vi "DATADYNINGELIANCE.vi"(6 "Channel":T2=enum."PCAN_USBBUS1", 7 "StepCMOD":u16(ring) items=["PostDCIR", "intraDCIR", "PreDCIR"], 8 "errin":errorcluster, 10 "L2T":T1 caption="Limites de test pris en compte", 11 "3P4S":bool) -> (0 "errout":errorcluster caption="sortie d'erreur", 1 "CAN TIME out":bool, 2 "Out":T4, 3 "test OK?":bool, 4 "cluster de sortie":T3)   [LabVIEW 2020]
doc: "Test les modules via la carte CMOD"
uses:
  <userlib>/PCAN Basic/Controls/Channel.ctl
  Ctrl/L2T.ctl
  <userlib>/PCAN Basic/Controls/BaudrateEenum.ctl
  <userlib>/Alex_Peak_lib/PEAK_lib_ALEX.lvlib
  <userlib>/PCAN Basic/PCANBasic.lvlib
panel:
  # "Pre DCIR_____________________________________"
  # "intra DCIR_____________________________________"
  # "Post DCIR_____________________________________"
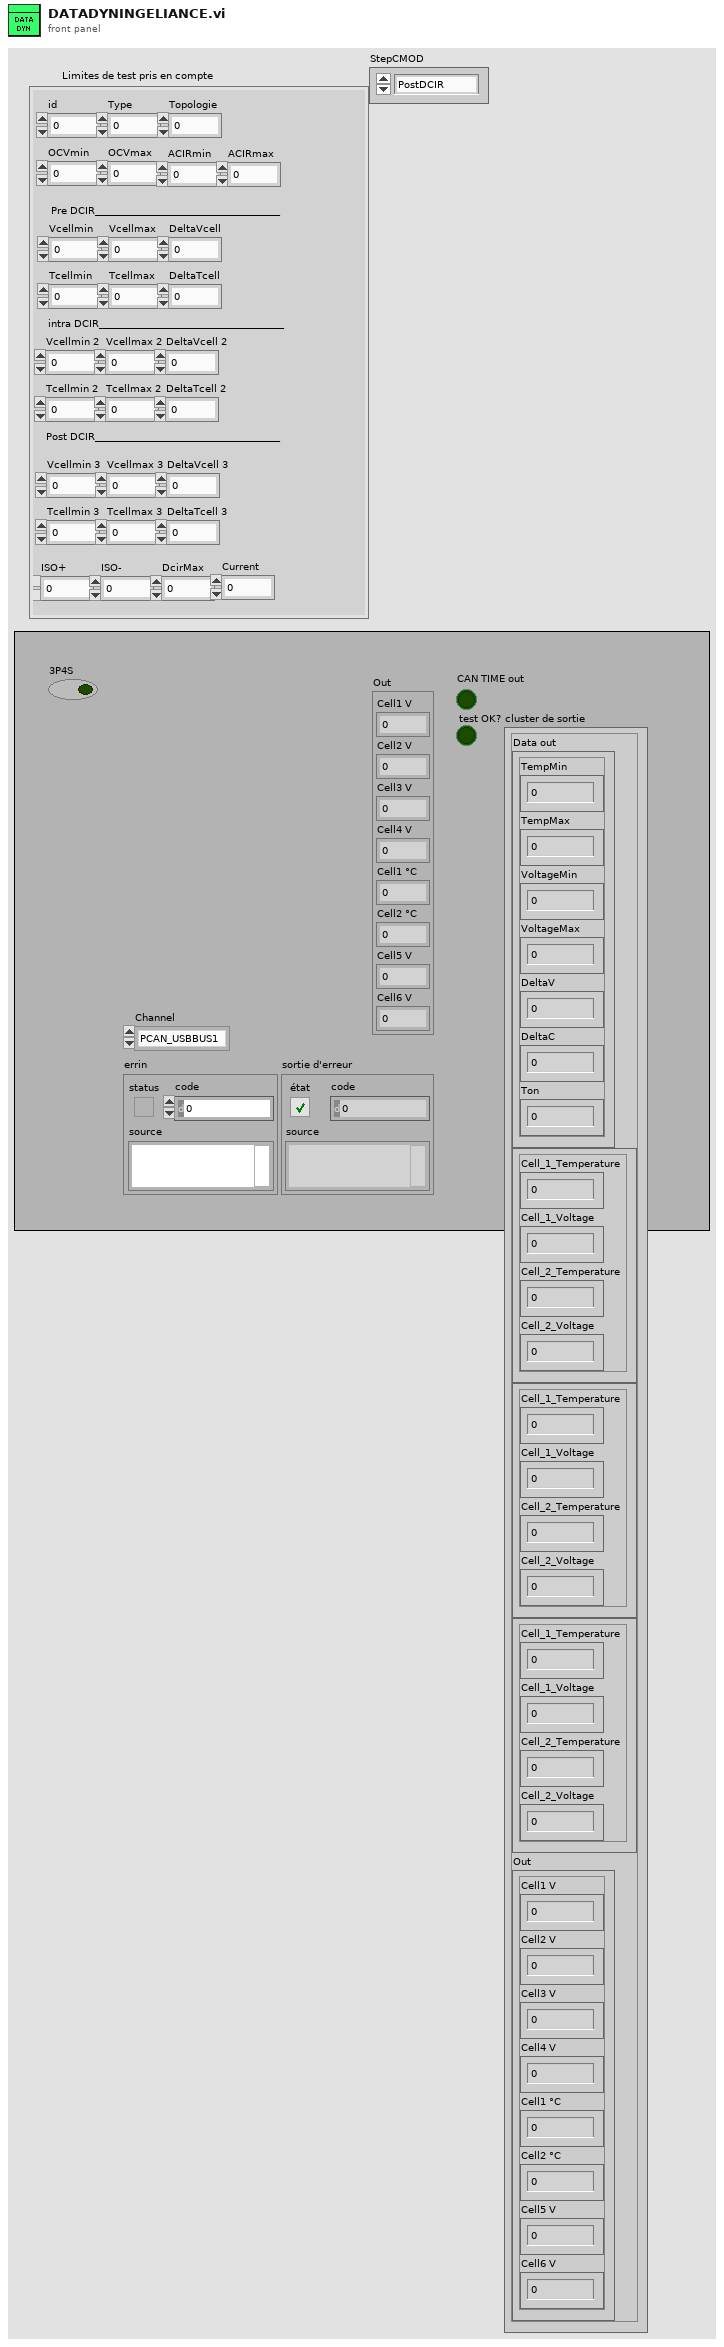
[diagram p1: front panel]
types:
  T1 = typedef "L2T.ctl" = cluster{"id":dbl, "Type":dbl, "OCVmin":dbl, "OCVmax":dbl, "ACIRmin":dbl, "ACIRmax":dbl, "Vcellmin":dbl, "Vcellmax":dbl, "DeltaVcell":dbl, "Tcellmin":dbl, "Tcellmax":dbl, "DeltaTcell":dbl, "ISO+":dbl, "ISO-":dbl, "DcirMax":dbl, "Current":dbl, "Topologie":dbl, "Vcellmin 2":dbl, "Vcellmax 2":dbl, "DeltaVcell 2":dbl, "Tcellmin 2":dbl, "Tcellmax 2":dbl, "DeltaTcell 2":dbl, "Vcellmin 3":dbl, "Vcellmax 3":dbl, "DeltaVcell 3":dbl, "Tcellmin 3":dbl, "Tcellmax 3":dbl, "DeltaTcell 3":dbl}
  T2 = typedef "PCANBasic.lvlib/Channel.ctl" = enum16{"PCAN_NONEBUS", "not used1", "not used2", "not used3", "not used4", "not used5", "not used6", "not used7", "not used8", "not used9", "not used10", "not used11", "not used12", "not used13", "not used14", "not used15", "not used16", "not used17", "not used18", "not used19", "not used20", "not used21", "not used22", "not used23", "not used24", "not used25", "not used26", "not used27", "not used28", "not used29", "not used30", "not used31", "not used32", "PCAN_ISABUS1", "PCAN_ISABUS2", "PCAN_ISABUS3", "PCAN_ISABUS4", "PCAN_ISABUS5", "PCAN_ISABUS6", "PCAN_ISABUS7", "PCAN_ISABUS8", "not used41", "not used42", "not used43", "not used44", "not used45", "not used46", "not used47", "not used48", "PCAN_DNGBUS1", "not used50", "not used51", "not used52", "not used53", "not used54", "not used55", "not used56", "not used57", "not used58", "not used59", "not used60", "not used61", "not used62", "not used63", "not used64", "PCAN_PCIBUS1", "PCAN_PCIBUS2", "PCAN_PCIBUS3", "PCAN_PCIBUS4", "PCAN_PCIBUS5", "PCAN_PCIBUS6", "PCAN_PCIBUS7", "PCAN_PCIBUS8", "not used73", "not used74", "not used75", "not used76", "not used77", "not used78", "not used79", "not used80", "PCAN_USBBUS1", "PCAN_USBBUS2", "PCAN_USBBUS3", "PCAN_USBBUS4", "PCAN_USBBUS5", "PCAN_USBBUS6", "PCAN_USBBUS7", "PCAN_USBBUS8", "Not used89", "Not used90", "Not used91", "Not used92", "Not used93", "Not used94", "Not used95", "Not used96", "PCAN_PCCBUS1", "PCAN_PCCBUS2"}
  T3 = cluster{"Data out":cluster{"TempMin":sgl, "TempMax":sgl, "VoltageMin":sgl, "VoltageMax":sgl, "DeltaV":sgl, "DeltaC":sgl, "Ton":sgl}, "Cluster":cluster{"Cell_1_Temperature":sgl, "Cell_1_Voltage":sgl, "Cell_2_Temperature":sgl, "Cell_2_Voltage":sgl}, "Cluster":cluster{"Cell_1_Temperature":sgl, "Cell_1_Voltage":sgl, "Cell_2_Temperature":sgl, "Cell_2_Voltage":sgl}, "Cluster":cluster{"Cell_1_Temperature":sgl, "Cell_1_Voltage":sgl, "Cell_2_Temperature":sgl, "Cell_2_Voltage":sgl}, "Out":cluster{"Cell1 V":sgl, "Cell2 V":sgl, "Cell3 V":sgl, "Cell4 V":sgl, "Cell1 °C":sgl, "Cell2 °C":sgl, "Cell5 V":sgl, "Cell6 V":sgl}}
  T4 = cluster{"Cell1 V":sgl, "Cell2 V":sgl, "Cell3 V":sgl, "Cell4 V":sgl, "Cell1 °C":sgl, "Cell2 °C":sgl, "Cell5 V":sgl, "Cell6 V":sgl}
  T5 = typedef "PCANBasic.lvlib/BaudrateEenum.ctl" = enum16{"CAN_Baud_1M", "CAN_Baud_800K", "CAN_BAUD_500K", "CAN_BAUD_250K", "CAN_BAUD_125K", "CAN_BAUD_100K", "CAN_BAUD_95K", "CAN_BAUD_83K", "CAN_BAUD_50K", "CAN_BAUD_47K", "CAN_BAUD_33K", "CAN_BAUD_20K", "CAN_BAUD_10K", "CAN_BAUD_5K", "User Baudrate"}
  T6 = cluster{"TempMin":sgl, "TempMax":sgl, "VoltageMin":sgl, "VoltageMax":sgl, "DeltaV":sgl, "DeltaC":sgl, "Ton":sgl}
  T7 = cluster{"Cell_1_Temperature":sgl, "Cell_1_Voltage":sgl, "Cell_2_Temperature":sgl, "Cell_2_Voltage":sgl}
  T8 = cluster{"ID":u32, "MSGTYPE":u8, "LEN":u8, "DATA[0]":u8, "DATA[1]":u8, "DATA[2]":u8, "DATA[3]":u8, "DATA[4]":u8, "DATA[5]":u8, "DATA[6]":u8, "DATA[7]":u8}
  T9 = cluster{"Cell1 V":string, "Cell2 V":string, "Cell3 V":string, "Cell4 V":string, "Cell1 °C":string, "Cell2 °C":string, "Cell5 V":string, "Cell6 V":string}
  T10 = cluster{"Data out":cluster{"TempMin":sgl, "TempMax":sgl, "VoltageMin":sgl, "VoltageMax":sgl, "DeltaV":sgl, "DeltaC":sgl, "Ton":sgl}, cluster{"Cell_1_Temperature":sgl, "Cell_1_Voltage":sgl, "Cell_2_Temperature":sgl, "Cell_2_Voltage":sgl}, cluster{"Cell_1_Temperature":sgl, "Cell_1_Voltage":sgl, "Cell_2_Temperature":sgl, "Cell_2_Voltage":sgl}, cluster{"Cell_1_Temperature":sgl, "Cell_1_Voltage":sgl, "Cell_2_Temperature":sgl, "Cell_2_Voltage":sgl}, "Out":cluster{"Cell1 V":sgl, "Cell2 V":sgl, "Cell3 V":sgl, "Cell4 V":sgl, "Cell1 °C":sgl, "Cell2 °C":sgl, "Cell5 V":sgl, "Cell6 V":sgl}}
  T11 = cluster{"millis":u32, "millis_overflow":u16, "micros":u16}
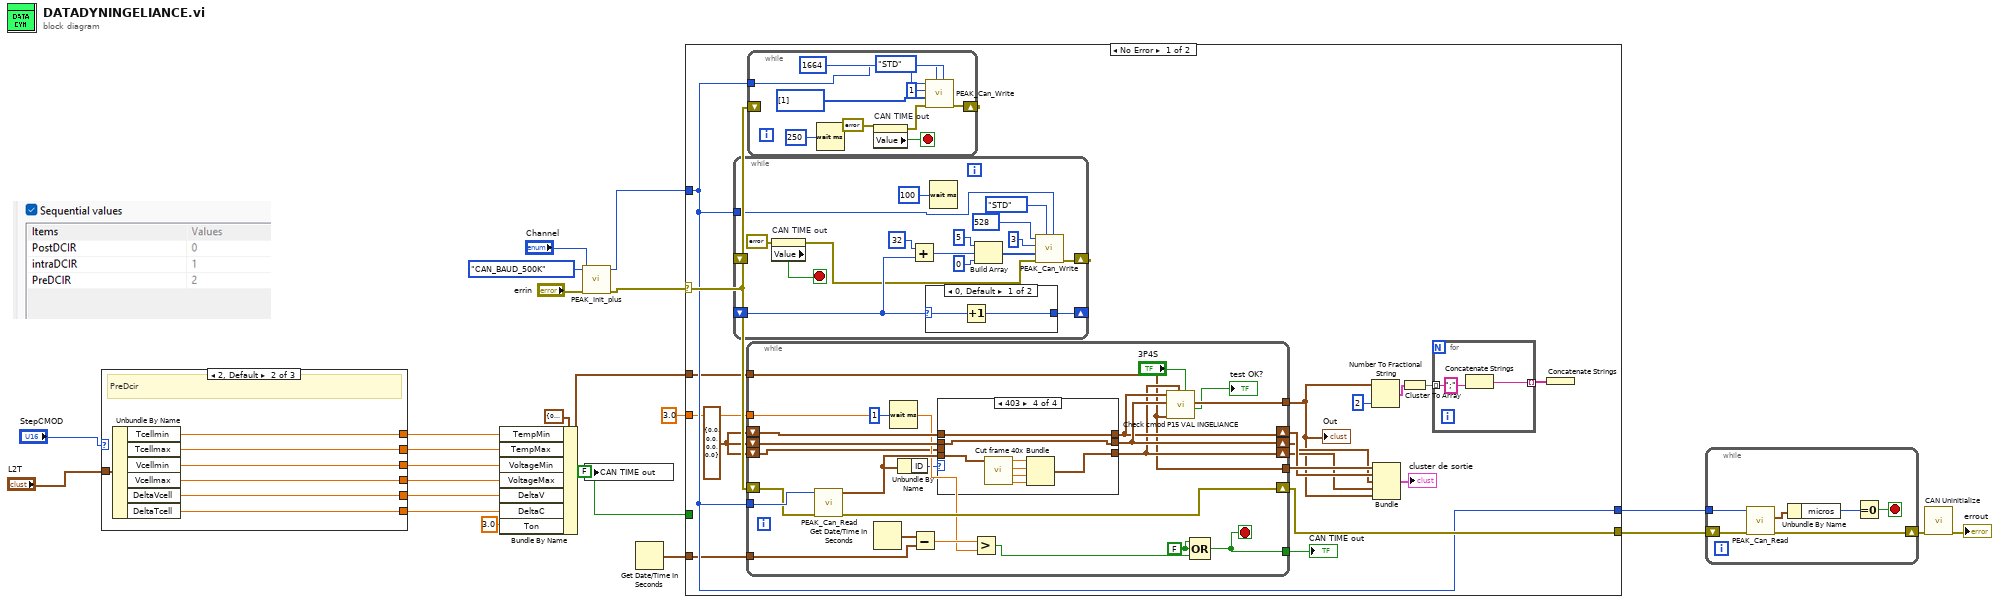
[diagram p0: block diagram]
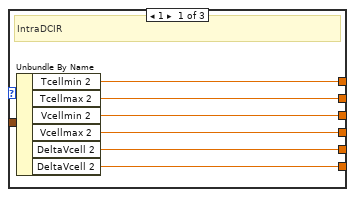
[diagram p2: hidden frame]
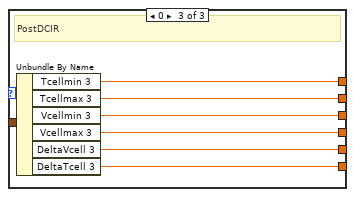
[diagram p3: hidden frame]
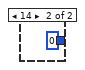
[diagram p4: hidden frame]
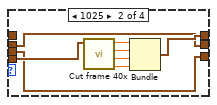
[diagram p6: hidden frame]
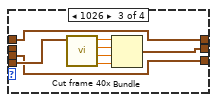
[diagram p7: hidden frame]
diagram:
  w21 = FALSE ("Booléen")
  n1 = case shown="2, Default" "StepCMOD" {
    tunnel: [w30 w37 w44] -> w14
    tunnel: [w29 w36 w43] -> w13
    tunnel: [w28 w35 w42] -> w12
    tunnel: [w27 w34 w41] -> w11
    tunnel: [w26 w33 w40] -> w10
    tunnel: [w25 w32 w39] -> w9
    tunnel: "L2T" -> [w24 w31 w38]
    frame 1 {
      # "IntraDCIR"
      n2 = Unbundle By Name(w24) -> ("Tcellmin 2"=w30:dbl, "Tcellmax 2"=w29:dbl, "Vcellmin 2"=w28:dbl, "Vcellmax 2"=w27:dbl, "DeltaVcell 2"=w26:dbl, "DeltaVcell 2"=w25:dbl)
    }
    frame 2, Default {
      # "PreDcir"
      n3 = Unbundle By Name(w31) -> ("Tcellmin"=w37:dbl, "Tcellmax"=w36:dbl, "Vcellmin"=w35:dbl, "Vcellmax"=w34:dbl, "DeltaVcell"=w33:dbl, "DeltaTcell"=w32:dbl)
    }
    frame 0 {
      # "PostDCIR"
      n4 = Unbundle By Name(w38) -> ("Tcellmin 3"=w44:dbl, "Tcellmax 3"=w43:dbl, "Vcellmin 3"=w42:dbl, "Vcellmax 3"=w41:dbl, "DeltaVcell 3"=w40:dbl, "DeltaTcell 3"=w39:dbl)
    }
  }
  n5 = Bundle By Name(cluster=T6 {"TempMin"=0.0, "TempMax"=0.0, "VoltageMin"=0.0, "VoltageMax"=0.0, "DeltaV"=0.0, "DeltaC"=0.0, "Ton"=0.0} ("Data out"), "TempMin"=w14, "TempMax"=w13, "VoltageMin"=w12, "VoltageMax"=w11, "DeltaV"=w10, "DeltaC"=w9, "Ton"=sgl 3.0) -> (w6:T6)
  n6 = call "PEAK_Init_plus.vi"("errin"="errin", "Channel"="Channel", "BTR0BTR1"=BaudrateEenum."CAN_BAUD_500K") -> ("errout"=w19:errorcluster, "Channel out"=w20:T2)  [unwired: 7 in]
  n7 = local write "CAN TIME out"(w21) -> ()
  n8 = Get Date/Time In Seconds() -> (seconds since 1Jan1904=w22:timestamp)
  n9 = case shown="No Error" w19 {
    selector: w19 -> [w62 w146]
    tunnel: w20 -> [w60 w145]
    tunnel: [w61 w146] -> w18
    tunnel: [w60 w145] -> w17
    tunnel: w22 -> [w58 _]
    tunnel: w6 -> [w57 _]
    tunnel: 3.0 ("Timeout") -> [w56 _]
    tunnel: w21 -> [_ _]
    frame No Error {
      w51 = T7 {"Cell_1_Temperature"=0.0, "Cell_1_Voltage"=0.0, "Cell_2_Temperature"=0.0, "Cell_2_Voltage"=0.0}
      n10 = while {
        tunnel: w60 -> [w76]
        shift-right: [w91] -> _
        shift-left: _ -> [w90]
        shift-right: [w89] -> _
        shift-left: w62 -> [_]
        stop <- w87 stop-if-true
        n11 = property on="CAN TIME out" class="Bool (strict)"(error in=errorcluster {"status"=FALSE, "code"=0, "source"=""} ("entrée d'erreur (pas d'erreur)")) -> (error out=w88:errorcluster, "Value"=w87:bool)  [unwired: 1 in, 1 out]
        n12 = Add(x=u8 32, y=w90) -> (x+y=w82:i32)
        n13 = case shown="0, Default" w90 {
          selector: w90 -> [w93 _]
          tunnel: [w92 0] -> w91
          frame 0, Default {
            n14 = Increment(x=w93) -> (x+1=w92:i32)
          }
          frame 14 {
          }
        }
        n15 = Wait (ms)(milliseconds to wait=u32 100 ("attente (ms)")) -> ()  [unwired: 1 out]
        n16 = Build Array(u8 5 ("élément"), w82, u8 0 ("élément")) -> (w81:i32[])
        n17 = call <userlib>:"PEAK_Can_Write.vi"("CAN Handle"=w76, "MSG type"=enum8{"STD", "RTR", "XTD", "XTD RTR", "STATUS"}."STD", "errin"=w88, "CAN Data"=w81, "DLC (8)"=u8 3, "Identifier"=u32 528) -> ("errout"=w89:errorcluster)  [unwired: 5 in]
      }
      n18 = while {
        shift-right: [w111] -> w61
        shift-left: w62 -> [w115]
        shift-right: [w109] -> w49
        shift-left: w51 -> [w113]
        shift-right: [w110] -> w48
        shift-left: w51 -> [w112]
        tunnel: w60 -> [w116]
        tunnel: [w108] -> w46
        tunnel: [w107] -> w59
        tunnel: w58 -> [w103]
        tunnel: w57 -> [w95]
        tunnel: w56 -> [w102]
        shift-right: [w98] -> w47
        shift-left: w51 -> [w101]
        tunnel: [w95] -> w50
        stop <- w107 stop-if-true
        w99 = FALSE ("valeur")
        n19 = call <userlib>:"PEAK_Can_Read.vi"("errin"=w115, "Channel out"=w116) -> ("errout"=w111:errorcluster, "MessageBuffer out"=w114:T8)  [unwired: 7 in, 1 out]
        n20 = Get Date/Time In Seconds() -> (seconds since 1Jan1904=w104:timestamp)
        n21 = Wait (ms)(milliseconds to wait=u32 1 ("attente (ms)")) -> ()  [unwired: 1 out]
        n22 = Unbundle By Name(w114) -> ("ID"=w100:u32)
        n23 = Subtract(x=w104, y=w103) -> (x-y=w105:dbl)
        n24 = case shown="403" w100 {
          tunnel: w114 -> [_ w123 w131 w140]
          tunnel: [w120 w124 w130 w138] -> w109
          tunnel: [w119 w122 w132 w137] -> w110
          tunnel: w113 -> [w120 _ w130 w138]
          tunnel: w112 -> [w119 w122 _ w137]
          tunnel: [w118 w121 w129 w139] -> w98
          tunnel: w101 -> [w118 w121 w129 _]
          frame 0, Default {
          }
          frame 1025 {
            n25 = call "Cut frame 40x.vi"("MessageBuffer out"=w123) -> ("Cell_2_Voltage"=w125:sgl, "Cell_2_Temperature"=w126:sgl, "Cell_1_Voltage"=w127:sgl, "Cell_1_Temperature"=w128:sgl)  [unwired: 7 in]
            n26 = Bundle("Cell_1_Temperature"=w128, "Cell_1_Voltage"=w127, "Cell_2_Temperature"=w126, "Cell_2_Voltage"=w125) -> (w124:T7)  [unwired: 1 in]
          }
          frame 1026 {
            n27 = call "Cut frame 40x.vi"("MessageBuffer out"=w131) -> ("Cell_2_Voltage"=w133:sgl, "Cell_2_Temperature"=w134:sgl, "Cell_1_Voltage"=w135:sgl, "Cell_1_Temperature"=w136:sgl)  [unwired: 7 in]
            n28 = Bundle("Cell_1_Temperature"=w136, "Cell_1_Voltage"=w135, "Cell_2_Temperature"=w134, "Cell_2_Voltage"=w133) -> (w132:T7)  [unwired: 1 in]
          }
          frame 1027 {
            n29 = call "Cut frame 40x.vi"("MessageBuffer out"=w140) -> ("Cell_2_Voltage"=w141:sgl, "Cell_2_Temperature"=w142:sgl, "Cell_1_Voltage"=w143:sgl, "Cell_1_Temperature"=w144:sgl)  [unwired: 7 in]
            n30 = Bundle("Cell_1_Temperature"=w144, "Cell_1_Voltage"=w143, "Cell_2_Temperature"=w142, "Cell_2_Voltage"=w141) -> (w139:T7)  [unwired: 1 in]
          }
        }
        n31 = Greater?(x=w105, y=w102) -> (0:w106:bool)
        n32 = call "Check cmod P15 VAL INGELIANCE.vi"("3P4S"="3P4S", "Cell 5 et 6"=w98, "Limites"=w95, "Cell 3 et 4"=w110, "Cell 1 et 2"=w109) -> ("ok global"=→"test OK?":bool, "Out"=w108:T4)  [unwired: 2 in, 3 out]
        n33 = Compound Arithmetic op=OR(w99, w99, w106) -> (w107:bool)
      }
      "CAN TIME out" <- w59
      "Out" <- w46
      n34 = while {
        tunnel: w60 -> [w68]
        shift-right: [w72] -> _
        shift-left: w62 -> [_]
        stop <- w75 stop-if-true
        n35 = Wait (ms)(milliseconds to wait=u32 250 ("attente (ms)")) -> ()  [unwired: 1 out]
        n36 = property on="CAN TIME out" class="Bool (strict)"(error in=errorcluster {"status"=FALSE, "code"=0, "source"=""} ("entrée d'erreur (pas d'erreur)")) -> (error out=w71:errorcluster, "Value"=w75:bool)  [unwired: 1 in, 1 out]
        n37 = call <userlib>:"PEAK_Can_Write.vi"("CAN Handle"=w68, "MSG type"=enum8{"STD", "RTR", "XTD", "XTD RTR", "STATUS"}."STD", "errin"=w71, "CAN Data"=u8[] [1], "DLC (8)"=u8 1, "Identifier"=u32 1664) -> ("errout"=w72:errorcluster)  [unwired: 5 in]
      }
      n38 = Number To Fractional String ("Nombre en chaîne fractionnaire")(number=w46, precision (6)=i16 2 ("précision (6)")) -> (F-format string=w54:T9)  [unwired: 2 in]
      n39 = Bundle("Data out"=w50, w49, w48, w47, "Out"=w46) -> (→"cluster de sortie":T10)  [unwired: 1 in]
      n40 = Cluster To Array(cluster=w54) -> (array=w53:string[])
      n41 = for {
        tunnel: w53 -> [w64] mode=indexing
        tunnel: [w63] -> w52 mode=indexing
        n42 = Concatenate Strings(w64, ";" ("chaîne")) -> (w63:string)
      }
      n43 = Concatenate Strings(w52) -> ()  [unwired: 1 out]
    }
    frame Error {
    }
  }
  n44 = while {
    tunnel: w17 -> [w151]
    shift-right: [w150] -> w16
    shift-left: w18 -> [w152]
    stop <- w148 stop-if-true
    n45 = call <userlib>:"PEAK_Can_Read.vi"("errin"=w152, "Channel out"=w151) -> ("errout"=w150:errorcluster, "TimestampBuffer out 2"=w147:T11)  [unwired: 7 in, 1 out]
    n46 = Unbundle By Name(w147) -> ("micros"=w149:u16)
    n47 = Equal To 0?(x=w149) -> (x = 0?=w148:bool)
  }
  n48 = call <userlib>:"CAN Uninitialize.vi"("error in (no error)"=w16) -> ("error out"=→"errout":errorcluster)  [unwired: 8 in, 2 out]
